vi "About ODE VI.vi"(10 "Model Name":string) -> ()   [LabVIEW 2014]
panel:
  out "About VI":string
  in  "Close":bool
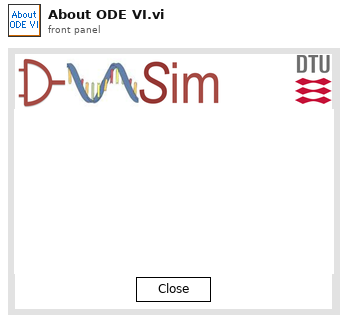
[diagram p1: front panel]
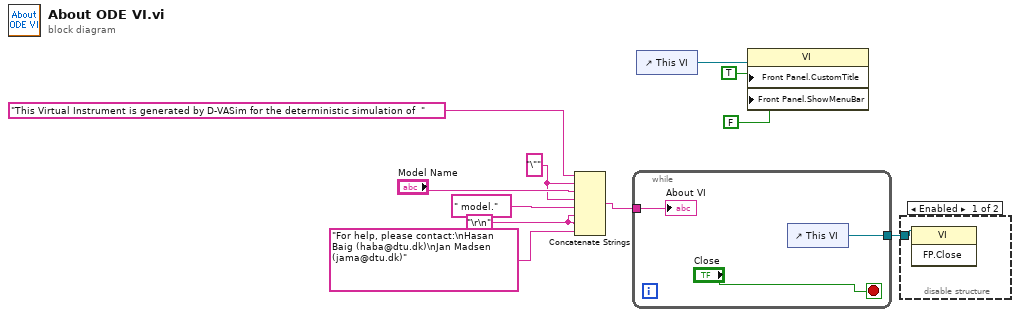
[diagram p0: block diagram]
diagram:
  w4 = "\r\n"
  w6 = "\"" ("string")
  n1 = Concatenate Strings("This Virtual Instrument is generated by D-VASim for the deterministic simulation of  ", w6, "Model Name", w6, " model." ("string"), w4, w4, "For help, please contact:\nHasan Baig (haba@dtu.dk)\nJan Madsen (jama@dtu.dk)" ("string")) -> (w2:string)
  n2 = while {
    tunnel: [w13] -> w11
    tunnel: w2 -> [w12]
    stop <- "Close" stop-if-true
    n3 = control-ref of="This VI"() -> (w13:refnum<vi>)
    "About VI" <- w12
  }
  n4 = control-ref of="This VI"() -> (w10:refnum<vi>)
  n5 = property class="VI"(reference=w10, "Front Panel.CustomTitle"=TRUE ("Front Panel Window:Custom Title"), "Front Panel.ShowMenuBar"=FALSE ("Front Panel Window:Show Menu Bar")) -> ()  [unwired: 1 in, 2 out]
  n6 = disable-structure shown="Enabled" {
    disable-tunnel: w11 -> [w15 _]
    frame Enabled {
      n7 = invoke class="VI" method="FP.Close"(reference=w15) -> ()  [unwired: 2 in, 3 out]
    }
    frame Disabled {
    }
  }
